vi "读取簇.vi"(8 "error in (no error)":errorcluster caption="错误输入（无错误）", 11 "VISA输入":refnum<class "VISA.lvclass">) -> (0 "error out":errorcluster caption="错误输出", 2 "簇":T1={"波特率"=9600, "数据比特"=8, "parity (0:none)"=0, "超时"=10000} {"parity (0:none)" items=["None", "Odd", "Even", "Mark", "Space"]}, 3 "VISA输出":refnum<class "VISA.lvclass">)   [LabVIEW 2016, in "VISA.lvclass"]
uses:
  VISA.lvclass
  VISA.lvclass/VISA.ctl
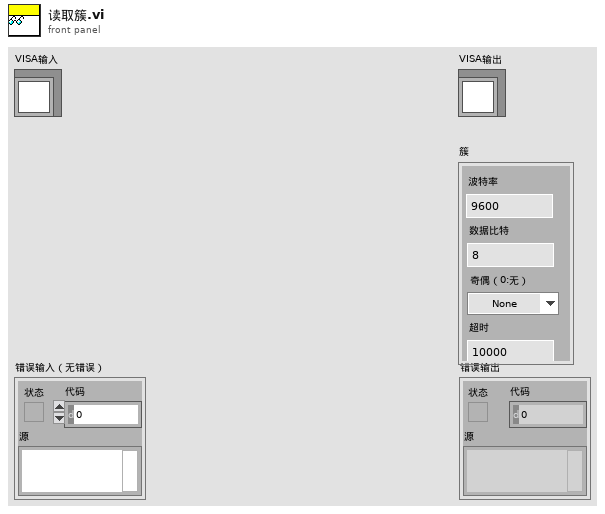
[diagram p1: front panel]
types:
  T1 = cluster{"波特率":u32, "数据比特":u16, "parity (0:none)":u16, "超时":u32}
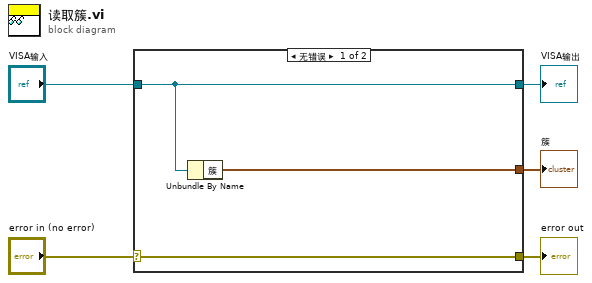
[diagram p0: block diagram]
diagram:
  n1 = case shown="无错误" "error in (no error)" {
    selector: "error in (no error)" -> [w8 w9]
    tunnel: [w8 w9] -> w4
    tunnel: [w7 w10] -> w2
    tunnel: "VISA输入" -> [w7 w10]
    tunnel: [w6 _] -> w1
    frame No Error {
      n2 = Unbundle By Name(w7) -> ("簇"=w6:T1)
    }
    frame Error {
    }
  }
  "error out" <- w4
  "VISA输出" <- w2
  "簇" <- w1
